vi "FPGA Open Reference.vi"(6 "max num IRQs":i32=1, 7 "Run?":T2, 8 "error in (no error)":errorcluster, 9 "Names of Registers":T1, 10 "FPGA Resource":string="RIO0", 11 "Bitfile Path":path) -> (0 "error out":errorcluster, 3 "FPGA Session":refnum<class "FPGA Interface Base.lvclass">)   [LabVIEW 2010, in "FPGA Interface Base.lvclass"]
uses:
  <userlib>/_FPGA Interface Advanced Tools/FPGA Interface Base/FPGA Interface Base.lvclass
  <userlib>/_FPGA Interface Advanced Tools/FPGA Interface Wrapper/TypeDefs/Open Attribute.ctl
  <userlib>/_FPGA Interface Advanced Tools/FPGA Interface Base/TypeDefs/FPGA Register Names.ctl
  <userlib>/_FPGA Interface Advanced Tools/FPGA Interface Wrapper/FPGA Interface Wrapper.lvlib
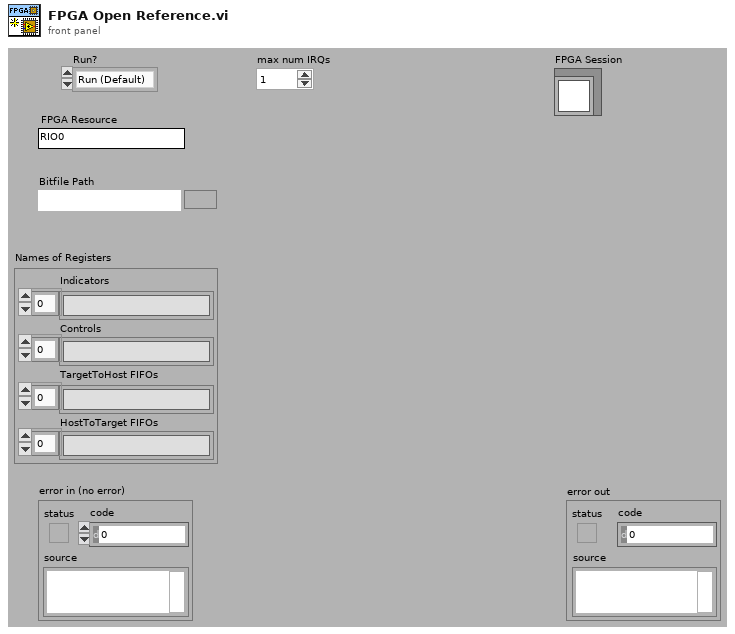
[diagram p1: front panel]
types:
  T1 = typedef "FPGA Interface Base.lvclass/FPGA Register Names.ctl" = cluster{"Indicators":string[], "Controls":string[], "TargetToHost FIFOs":string[], "HostToTarget FIFOs":string[]}
  T2 = typedef "FPGA Interface Wrapper.lvlib/Open Attribute.ctl" = enum32{"Run (Default)", "No Run"}
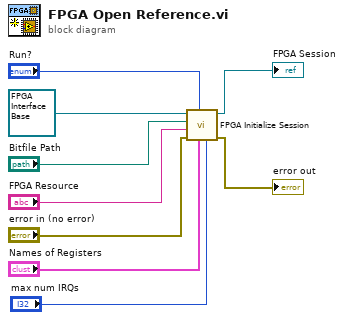
[diagram p0: block diagram]
diagram:
  n1 = call-dynamic "FPGA Initialize Session.vi"("max num IRQs"="max num IRQs", "Names of Registers"="Names of Registers", "Run?"="Run?", "error in (no error)"="error in (no error)", "FPGA Resource"="FPGA Resource", "Bitfile Path"="Bitfile Path", "FPGA Interface Base In"=refnum<class "FPGA Interface Base.lvclass"> refnum ("FPGA Interface Base.lvclass")) -> ("error out"=→"error out":errorcluster, "FPGA Interface Base Out"=→"FPGA Session":refnum<class "FPGA Interface Base.lvclass">)  [unwired: 3 in]
